vi "AM_Modulation.vi"(4 "Fs":dbl, 6 "Fc":dbl, 10 "message":dbl[](array[numeric])) -> (2 "mod_signal":dbl[](array[numeric]))   [LabVIEW 2011]
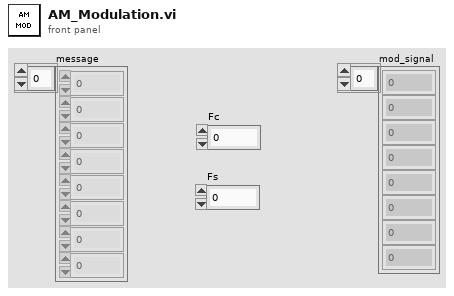
[diagram p1: front panel]
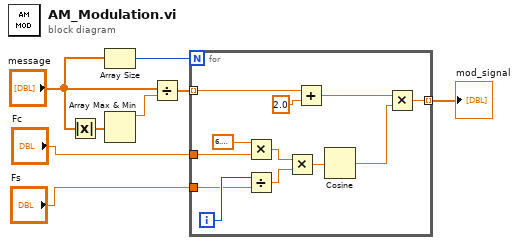
[diagram p0: block diagram]
diagram:
  n1 = Absolute Value(x="message") -> (abs(x)=w7:dbl[])
  n2 = Array Size(array="message") -> (size(s)=w8:i32)
  n3 = Array Max & Min(array=w7) -> (max value=w6:dbl)  [unwired: 3 out]
  n4 = Divide(x="message", y=w6) -> (x/y=w5:dbl[])
  n5 = for {
    N: w8 -> [_]
    tunnel: w5 -> [w11] mode=indexing
    tunnel: "Fc" -> [w19]
    tunnel: "Fs" -> [w17]
    tunnel: [w12] -> w1 mode=indexing
    i -> [w18]
    n6 = Multiply(x=6.283185307179586, y=w19) -> (x*y=w16:dbl)
    n7 = Divide(x=w18, y=w17) -> (x/y=w15:dbl)
    n8 = Multiply(x=w16, y=w15) -> (x*y=w14:dbl)
    n9 = Add(x=w11, y=2.0) -> (x+y=w10:dbl)
    n10 = Cosine(x=w14) -> (cos(x)=w13:dbl)
    n11 = Multiply(x=w10, y=w13) -> (x*y=w12:dbl)
  }
  "mod_signal" <- w1
